vi "IPC-Modbus-Transfer-EncodeResponse-Exceptions.vi"(10 "错误码":u8, 11 "功能码":u8) -> (3 "输出字符串":string)   [LabVIEW 2014]
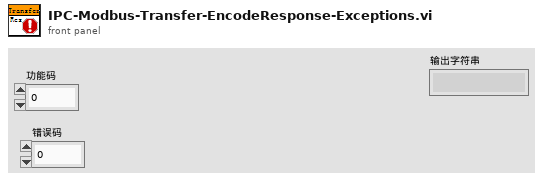
[diagram p1: front panel]
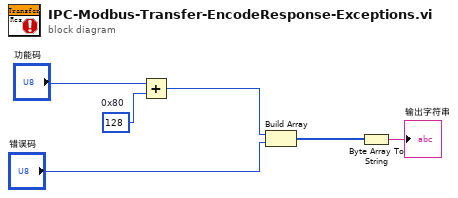
[diagram p0: block diagram]
diagram:
  w5 = u8 128  # 0x80
  n1 = Add(x="功能码", y=w5) -> (x+y=w4:u8)
  n2 = Build Array(w4, "错误码") -> (w2:u8[])
  n3 = Byte Array To String(unsigned byte array=w2) -> (string=→"输出字符串":string)
